vi "Streaming Example.vi"() -> ()   [LabVIEW 2020]
uses:
  g_industrial_cam/Device Enumeration.ctl
  g_industrial_cam/Camera/Camera.lvclass/Camera.ctl
  g_industrial_cam/Buffer/Buffer.lvclass/Buffer.ctl
  g_industrial_cam/Camera/GetSetPixelFormat.vi
  g_industrial_cam/Buffer/Access Handle.vi
  g_industrial_cam/Buffer/Read Data.vi
  g_industrial_cam/Buffer/Read Data as Mono8 Image.vi
  g_industrial_cam/Buffer/Read Data as Mono10 Image.vi
  g_industrial_cam/Buffer/Read Data as Mono10p Image.vi
  g_industrial_cam/Buffer/Read Data as Mono12 Image.vi
  g_industrial_cam/Buffer/Read Data as Mono12p Image.vi
  g_industrial_cam/Buffer/Read Data as Mono14 Image.vi
  g_industrial_cam/Buffer/Read Data as Mono14p Image.vi
  g_industrial_cam/Buffer/Read Data as Mono16 Image.vi
  g_industrial_cam/Buffer/Draw to Picture.vi
  g_industrial_cam/Buffer/Draw RGB8 to Picture.vi
  g_industrial_cam/Buffer/Draw BGR8 to Picture.vi
  g_industrial_cam/Buffer/ReadDataAsMono2Byte.vi
  g_industrial_cam/Buffer/DrawToPictureCore.vi
  g_industrial_cam/Camera/Check Not Disconnected.vi
  <vilib>/Utility/error.llb/Error Cluster From Error Code.vi
  g_industrial_cam/Camera/Destroy Stream Events.vi
  g_industrial_cam/Camera/Check Stream OK.vi
  <vilib>/picture/picture.llb/Draw Unflattened Pixmap.vi
  <vilib>/picture/picture.llb/Draw 8-Bit Pixmap.vi
  g_industrial_cam/Buffer/Buffer.lvclass
  g_industrial_cam/Camera/Camera.lvclass
panel:
  out "Pixel Formats":string[](array[string])
  out "Frame-Error Count":u64
  out "Frame Count (inc Errors)":u64
  out "Timeout":bool
  out "Devices":T1[](array[typedef])
  in  "Picture Zoom Factor":sgl
  out "Picture":picture
  in  "stop":bool
  out "error out":errorcluster
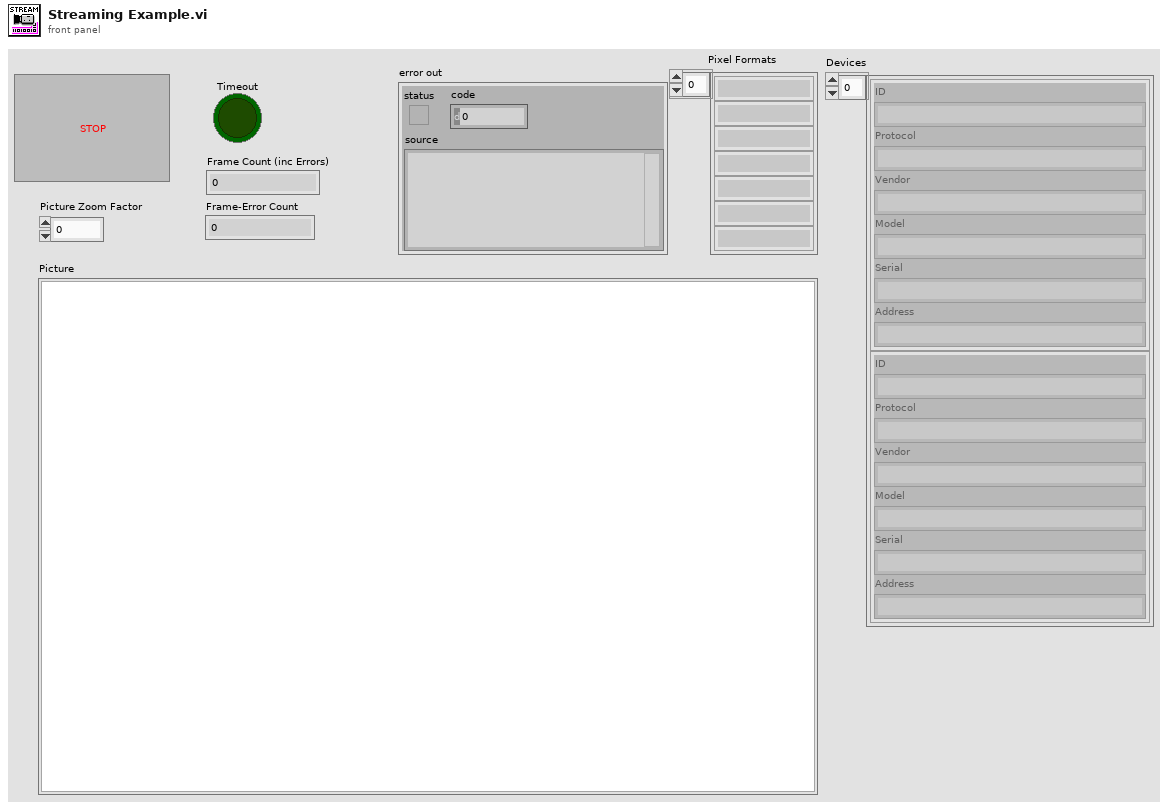
[diagram p1: front panel]
types:
  T1 = typedef "Device Enumeration.ctl" = cluster{"ID":string, "Protocol":string, "Vendor":string, "Model":string, "Serial":string, "Address":string}
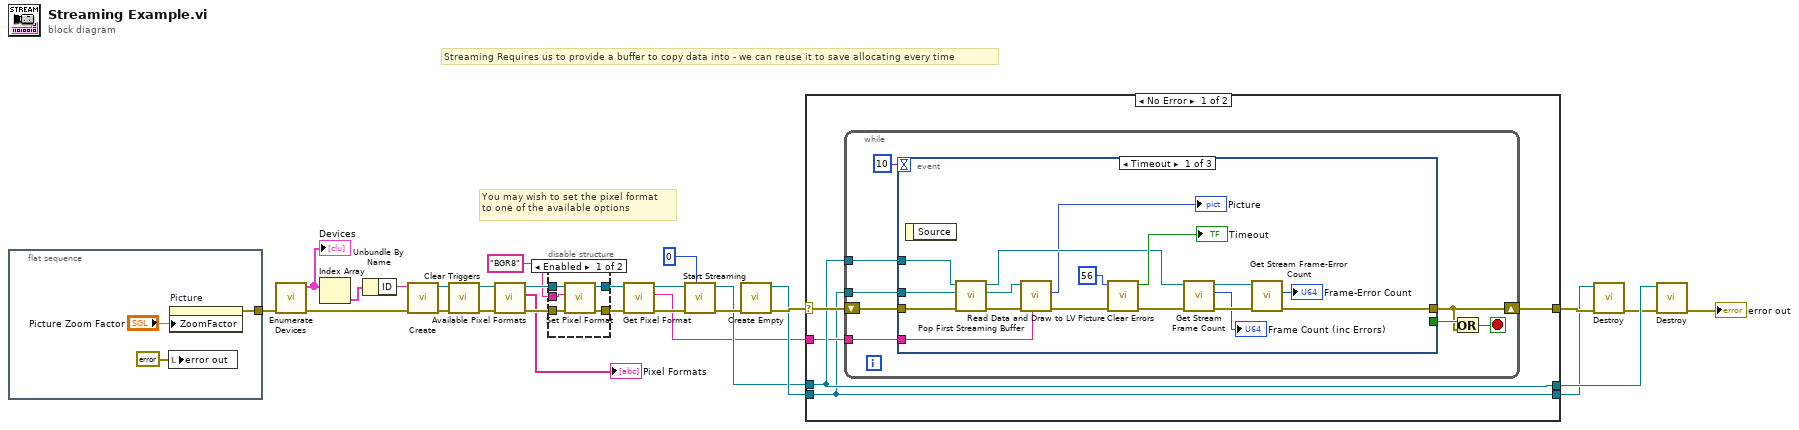
[diagram p0: block diagram]
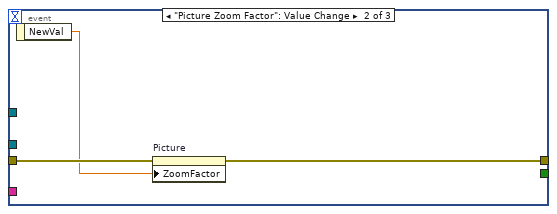
[diagram p3: hidden frame]
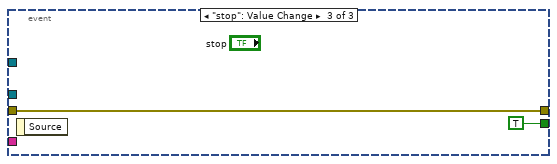
[diagram p4: hidden frame]
diagram:
  # "You may wish to set the pixel format\nto one of the available options"
  # "Streaming Requires us to provide a buffer to copy data into - we can reuse it to save allocating every time"
  n1 = flat-sequence {
    tunnel: [w31] -> w23
    frame #0 {
      n2 = local write "error out"(errorcluster {"status"=FALSE, "code"=0, "source"=""} ("error out")) -> ()
      n3 = property on="Picture" class="Pict"("ZoomFactor"="Picture Zoom Factor") -> (error out=w31:errorcluster)  [unwired: 2 in, 1 out]
    }
  }
  n4 = call "Enumerate Devices.vi"("error in (no error)"=w23) -> ("error out"=w26:errorcluster, "Devices"=w28:T1[])  [unwired: 9 in]
  "Devices" <- w28
  n5 = Index Array(array=w28) -> (element=w27:T1)  [unwired: 1 in]
  n6 = Unbundle By Name(w27) -> ("ID"=w25:string)
  n7 = call "Create.vi"("error in (no error)"=w26, "Identifier (ID, IP etc)"=w25) -> ("error out"=w24:errorcluster, "Camera"=w19:refnum<class "Camera.lvclass">)  [unwired: 8 in]
  n8 = call "Clear Triggers.vi"("error in (no error)"=w24, "Camera in"=w19) -> ("error out"=w14:errorcluster, "Camera"=w7:refnum<class "Camera.lvclass">)  [unwired: 8 in]
  n9 = call "Available Pixel Formats.vi"("error in (no error)"=w14, "Camera in"=w7) -> ("error out"=w8:errorcluster, "Pixel Formats"=→"Pixel Formats":string[], "Camera"=w4:refnum<class "Camera.lvclass">)  [unwired: 7 in]
  n10 = disable-structure shown="Enabled" {
    disable-tunnel: w8 -> [w36 w37]
    disable-tunnel: [w35 w37] -> w5
    disable-tunnel: w4 -> [w34 w38]
    disable-tunnel: [w33 w38] -> w3
    disable-tunnel: "BGR8" ("Pixel Format") -> [w32 _]
    frame Enabled {
      n11 = call "Set Pixel Format.vi"("error in (no error)"=w36, "Pixel Format"=w32, "Camera in"=w34) -> ("error out"=w35:errorcluster, "Camera"=w33:refnum<class "Camera.lvclass">)  [unwired: 7 in]
    }
    frame Disabled {
    }
  }
  n12 = call "Get Pixel Format.vi"("error in (no error)"=w5, "Camera in"=w3) -> ("error out"=w16:errorcluster, "Pixel Format"=w12:string, "Camera"=w15:refnum<class "Camera.lvclass">)  [unwired: 7 in]
  n13 = call "Start Streaming.vi"("Additional Buffers (Default: 3)"=u16 0, "error in (no error)"=w16, "Camera in"=w15) -> ("error out"=w22:errorcluster, "Camera"=w13:refnum<class "Camera.lvclass">)  [unwired: 7 in]
  n14 = call "Create Empty.vi"("error in (no error)"=w22) -> ("error out"=w21:errorcluster, "Empty Buffer"=w20:refnum<class "Buffer.lvclass">)  [unwired: 9 in]
  n15 = case shown="No Error" w21 {
    selector: w21 -> [w43 w75]
    tunnel: w13 -> [w41 w76]
    tunnel: [w42 w75] -> w11
    tunnel: [w41 w76] -> w18
    tunnel: w20 -> [w39 w74]
    tunnel: w12 -> [w40 _]
    tunnel: [w39 w74] -> w9
    frame No Error {
      n16 = while {
        shift-right: [w48] -> w42
        shift-left: w43 -> [w47]
        tunnel: w41 -> [w51]
        tunnel: w40 -> [w45]
        tunnel: w39 -> [w44]
        stop <- w49 stop-if-true
        n17 = event shown="[0] Timeout" {
          selector: _ -> [_ _ _]
          dyn-events: _ -> [_ _ _]
          timeout: 10 -> [_ _ _]
          tunnel: w51 -> [w68 _ _]
          tunnel: w47 -> [w67 w71 w73]
          tunnel: [w63 w70 w73] -> w48
          tunnel: [_ _ TRUE] -> w50
          tunnel: w45 -> [w54 _ _]
          tunnel: w44 -> [w52 _ _]
          event Timeout {
            n18 = event-data() -> ()  [unwired: 1 in, 1 out]
            n19 = call "Pop First Streaming Buffer.vi"("error in (no error)"=w67, "Buffer in"=w52, "Camera in"=w68) -> ("error out"=w58:errorcluster, "Buffer"=w56:refnum<class "Buffer.lvclass">, "Camera"=w55:refnum<class "Camera.lvclass">)  [unwired: 6 in]
            n20 = call "Read Data and Draw to LV Picture.vi"("Pixel Format"=w54, "error in (no error)"=w58, "Buffer in"=w56) -> ("error out"=w57:errorcluster, "Picture"=→"Picture":picture)  [unwired: 6 in, 1 out]
            n21 = call <vilib>:"Clear Errors.vi"("error in (no error)"=w57, "specific error code to clear (0: all)"=56) -> ("error out"=w66:errorcluster, "specific error cleared?"=→"Timeout":bool)  [unwired: 4 in]
            n22 = call "Get Stream Frame Count.vi"("error in (no error)"=w66, "Camera in"=w55) -> ("error out"=w62:errorcluster, "Frame Count (inc Errors)"=→"Frame Count (inc Errors)":u64, "Camera"=w61:refnum<class "Camera.lvclass">)  [unwired: 7 in]
            n23 = call "Get Stream Frame-Error Count.vi"("error in (no error)"=w62, "Camera in"=w61) -> ("error out"=w63:errorcluster, "Frame-Error Count"=→"Frame-Error Count":u64)  [unwired: 7 in, 1 out]
          }
          event "Picture Zoom Factor": Value Change {
            n24 = event-data() -> ("NewVal"=w69:sgl)  [unwired: 1 in]
            n25 = property on="Picture" class="Pict"(error in=w71, "ZoomFactor"=w69) -> (error out=w70:errorcluster)  [unwired: 1 in, 1 out]
          }
          event "stop": Value Change {
            n26 = event-data() -> ()  [unwired: 1 in, 1 out]
          }
        }
        n27 = Or(x=w50, y=w48) -> (x .or. y?=w49:bool)
      }
    }
    frame Error {
    }
  }
  n28 = call "Destroy.vi"("error in (no error)"=w11, "Buffer in"=w9) -> ("error out"=w10:errorcluster)  [unwired: 9 in]
  n29 = call "Destroy.vi"("error in (no error)"=w10, "Camera in"=w18) -> ("error out"=→"error out":errorcluster)  [unwired: 9 in]
